vi "test - save temp-Params to the top INI.vi"(8 "error in (no error)":errorcluster, 11 "TestCase in":refnum<class "csm-ini-variable-addon.lvclass">) -> (0 "error out":errorcluster, 3 "TestCase out":refnum<class "csm-ini-variable-addon.lvclass">)   [LabVIEW 2017, in "csm-ini-variable-addon.lvclass"]
uses:
  csm-ini-variable-addon.lvclass
  9da69169-e459-4de5-bd52-65d5bd10cfe3.vi
  819d10de-cc93-4901-8476-a53ff0da62fe.vi
  4331c652-d221-4445-b443-08c445718bf9.vi
  9da69169-e459-4de5-bd52-65d5bd10cfe3.vi/046f8cdf-7ef9-4292-8f14-7e46221fe55b.vi
  <vilib>/Utility/error.llb/Clear Errors.vi
  819d10de-cc93-4901-8476-a53ff0da62fe.vi/af4ed662-a05f-49e7-a783-9e8c565b17bc.vi
  4331c652-d221-4445-b443-08c445718bf9.vi/ed1a4760-8b7c-48d0-918c-41a9248c1a9b.vi
  <vilib>/Utility/Data Type/Get Type Information.vi
  <userlib>/_NEVSTOP/Communicable State Machine(CSM)/addons/API-String-Arugments-Support/_Support/Data To SingleElementsArray_csm.vi
  <userlib>/_NEVSTOP/Communicable State Machine(CSM)/addons/API-String-Arugments-Support/_Support/Data To API String Arguments.vi
  INI-Static-Variable-Support/_Support/Parse Used Session and Name.vi
  INI-Static-Variable-Support/_Support/INI-FGV.vi
  INI-Static-Variable-Support/_Support/global-csm-ini-db-change-flag.vi
  <userlib>/_NEVSTOP/Communicable State Machine(CSM)/addons/API-String-Arugments-Support/_Support/Convert API String Arguments to Data(variant).vi
  <userlib>/_NEVSTOP/Communicable State Machine(CSM)/addons/API-String-Arugments-Support/_Support/SingleElementsArray To Data_csm.vi
  INI-Static-Variable-Support/INI-Static-Variable-Support.lvlib
panel:
  out "config out":cluster{"Key":i32}
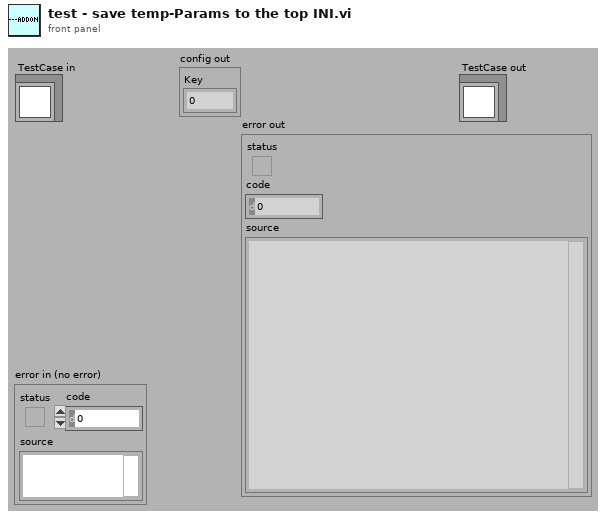
[diagram p1: front panel]
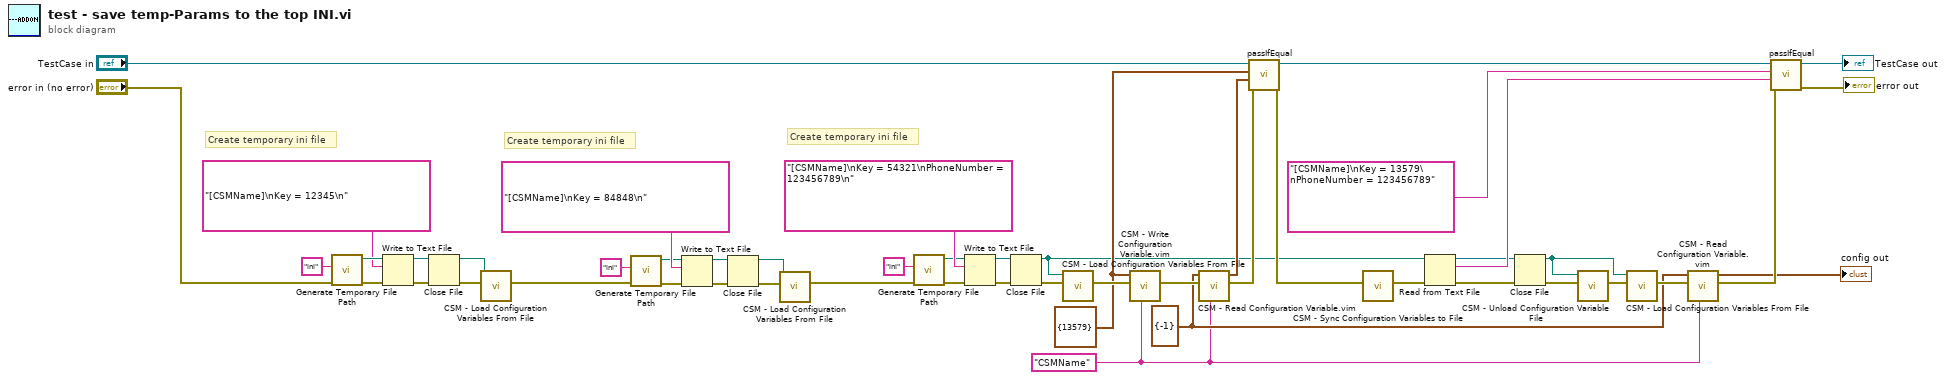
[diagram p0: block diagram]
diagram:
  w4 = cluster{"Key":i32} {"Key"=-1}
  w26 = cluster{"Key":i32} {"Key"=13579}
  w3 = "CSMName" ("Section Name(\"\" as Default)")
  # "Create temporary ini file"
  # "Create temporary ini file"
  # "Create temporary ini file"
  n1 = call <vilib>:"Generate Temporary File Path.vi"("error in (no error)"="error in (no error)", "Temporary File Extension (tmp)"="ini") -> ("error out"=w47:errorcluster, "Unique Temporary File Path"=w44:path)  [unwired: 8 in]
  n2 = Write to Text File(file (use dialog)=w44, text="[CSMName]\nKey = 12345\n", error in=w47) -> (refnum out=w43:refnum<file>, error out=w45:errorcluster)  [unwired: 1 in, 1 out]
  n3 = Close File(refnum=w43, error in=w45) -> (path=w21:path, error out=w42:errorcluster)
  n4 = call "CSM - Load Configuration Variables From File.vi"("error in (no error)"=w42, "Path"=w21) -> ("error out"=w10:errorcluster)  [unwired: 7 in]
  n5 = call <vilib>:"Generate Temporary File Path.vi"("error in (no error)"=w10, "Temporary File Extension (tmp)"="ini") -> ("error out"=w11:errorcluster, "Unique Temporary File Path"=w14:path)  [unwired: 8 in]
  n6 = Write to Text File(file (use dialog)=w14, text="[CSMName]\nKey = 84848\n", error in=w11) -> (refnum out=w15:refnum<file>, error out=w13:errorcluster)  [unwired: 1 in, 1 out]
  n7 = Close File(refnum=w15, error in=w13) -> (path=w18:path, error out=w16:errorcluster)
  n8 = call "CSM - Load Configuration Variables From File.vi"("error in (no error)"=w16, "Path"=w18) -> ("error out"=w9:errorcluster)  [unwired: 7 in]
  n9 = call <vilib>:"Generate Temporary File Path.vi"("error in (no error)"=w9, "Temporary File Extension (tmp)"="ini") -> ("error out"=w34:errorcluster, "Unique Temporary File Path"=w37:path)  [unwired: 8 in]
  n10 = Write to Text File(file (use dialog)=w37, text="[CSMName]\nKey = 54321\nPhoneNumber = 123456789\n", error in=w34) -> (refnum out=w38:refnum<file>, error out=w36:errorcluster)  [unwired: 1 in, 1 out]
  n11 = Close File(refnum=w38, error in=w36) -> (path=w22:path, error out=w39:errorcluster)
  n12 = call "CSM - Load Configuration Variables From File.vi"("error in (no error)"=w39, "Path"=w22) -> ("error out"=w33:errorcluster)  [unwired: 7 in]
  n13 = call "CSM - Write Configuration Variable.vim"("Section Name(\"\" as Default)"=w3, "error in (no error)"=w33, "Variant"=w26) -> ("error out"=w29:errorcluster)  [unwired: 5 in, 1 out]
  n14 = call "CSM - Read Configuration Variable.vim"("Section Name(\"\" as Default)"=w3, "error in (no error)"=w29, "config prototype(Cluster Prefered)"=w4) -> ("error out"=w24:errorcluster, "config out"=w25:cluster{"Key":i32})  [unwired: 5 in]
  n15 = call-dynamic "passIfEqual.vi"("error in (no error)"=w24, "y"=w25, "x"=w26, "TestCase in"="TestCase in") -> ("error out"=w23:errorcluster, "TestCase out"=w27:refnum<class "csm-ini-variable-addon.lvclass">)  [unwired: 6 in]
  n16 = call "CSM - Sync Configuration Variables to File.vi"("error in (no error)"=w23) -> ("error out"=w32:errorcluster)  [unwired: 8 in]
  n17 = Read from Text File(file (use dialog)=w22, error in=w32) -> (refnum out=w20:refnum<file>, text=w31:string, error out=w19:errorcluster)  [unwired: 2 in, 1 out]
  n18 = Close File(refnum=w20, error in=w19) -> (path=w6:path, error out=w8:errorcluster)
  n19 = call "CSM - Unload Configuration Variable File.vi"("error in (no error)"=w8, "Path"=w6) -> ("error out"=w7:errorcluster)  [unwired: 7 in]
  n20 = call "CSM - Load Configuration Variables From File.vi"("error in (no error)"=w7, "Path"=w6) -> ("error out"=w5:errorcluster)  [unwired: 7 in]
  n21 = call "CSM - Read Configuration Variable.vim"("Section Name(\"\" as Default)"=w3, "error in (no error)"=w5, "config prototype(Cluster Prefered)"=w4) -> ("error out"=w2:errorcluster, "config out"=→"config out":cluster{"Key":i32})  [unwired: 5 in]
  n22 = call-dynamic "passIfEqual.vi"("error in (no error)"=w2, "y"=w31, "x"="[CSMName]\nKey = 13579\nPhoneNumber = 123456789", "TestCase in"=w27) -> ("error out"=→"error out":errorcluster, "TestCase out"=→"TestCase out":refnum<class "csm-ini-variable-addon.lvclass">)  [unwired: 6 in]
